vi "RSZVB Set Electrical Length.vi"(7 "Electrical Length (0.0 m)":dbl format="%^.3e", 8 "error in (no error)":errorcluster {"code" format="%.0x"}, 9 "Port (1)":i32=1, 10 "Channel (1)":i32=1, 11 "VISA session":refnum<visa-resource-name>) -> (0 "error out":errorcluster {"code" format="%.0x"}, 3 "dup VISA session":refnum<visa-resource-name>)   [LabVIEW 2011]
doc: "This VI defines the offset parameter for test port <Port> as an electrical length.\n\nNote(s):\n\nRemote-control command(s):\n[SENSe<Ch>:]CORRection:EDELay<port_no>:ELENgth"
uses:
  _utility/RSZVB Global Data.vi
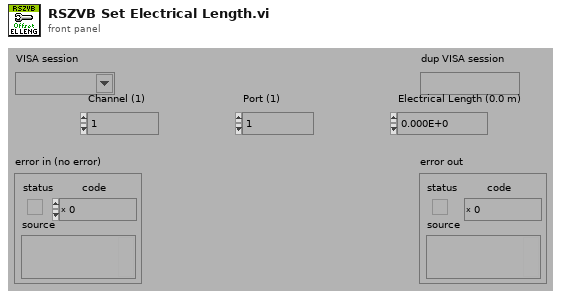
[diagram p1: front panel]
types:
  T1 = cluster{"Error Checking (T: On)":bool, "Installed Options":string[], "Data Valid?":bool, "Ports":i32, "Model":string[], "Option Checking (T: On)":bool}[]
  T2 = cluster{"Error Checking (T: On)":bool, "Installed Options":string[], "Data Valid?":bool, "Ports":i32, "Model":string[], "Option Checking (T: On)":bool}
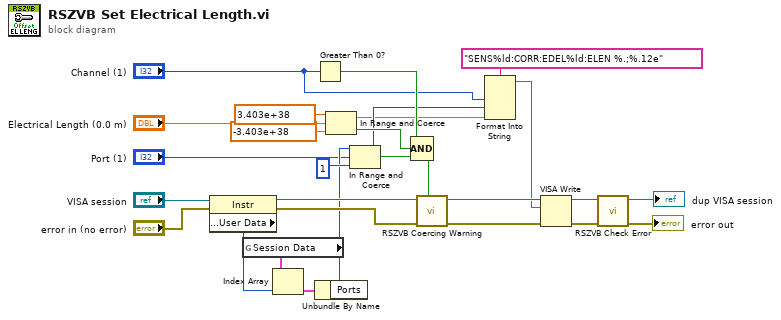
[diagram p0: block diagram]
diagram:
  n1 = property class="Instr"(reference="VISA session", error in="error in (no error)") -> (reference out=w16:refnum<visa-resource-name>, error out=w17:errorcluster, "General Settings:User Data"=w18:u32)
  n2 = global read "RSZVB Global Data.vi" "Session Data"() -> (w19:T1)
  n3 = Index Array(array=w19, index=w18) -> (element=w20:T2)
  n4 = Greater Than 0?(x="Channel (1)") -> (x > 0?=w21:bool)
  n5 = Unbundle By Name(w20) -> ("Ports"=w13:i32)
  n6 = In Range and Coerce(upper limit=3.403e+38, x="Electrical Length (0.0 m)", lower limit=-3.403e+38) -> (coerced(x)=w1:dbl, In Range?=w4:bool)
  n7 = In Range and Coerce(upper limit=w13, x="Port (1)", lower limit=1) -> (coerced(x)=w2:i32, In Range?=w14:bool)
  n8 = Compound Arithmetic op=AND(w21, w4, w14) -> (w23:bool)
  n9 = call "RSZVB Coercing Warning.vi"("In Range?"=w23, "error in (no error)"=w17, "VISA session"=w16) -> ("error out"=w26:errorcluster, "dup VISA session"=w27:refnum<visa-resource-name>)  [unwired: 7 in]
  n10 = Format Into String(format string="SENS%ld:CORR:EDEL%ld:ELEN %.;%.12e", "Channel (1)", w2, w1) -> (resulting string=w22:string)  [unwired: 2 in, 1 out]
  n11 = VISA Write(VISA resource name=w27, write buffer=w22, error in (no error)=w26) -> (VISA resource name out=w24:refnum<visa-resource-name>, error out=w25:errorcluster)  [unwired: 1 out]
  n12 = call "RSZVB Check Error.vi"("error in (no error)"=w25, "VISA session"=w24) -> ("error out"=→"error out":errorcluster, "dup VISA session"=→"dup VISA session":refnum<visa-resource-name>)  [unwired: 8 in]
